vi "nanocal publish -- frontpanel.vi"(7 "publisher action":T3, 10 "nanocal data array IN":T1[](array[typedef])) -> (2 "nanocal data array OUT":T1[](array[typedef]))   [LabVIEW 2018]
uses:
  publisher action.ctl
  icicle.ctl
  nanocal-frontend -- data type.ctl
panel:
  out "nanocal data OUT":T2
  in  "nanocal data":T2
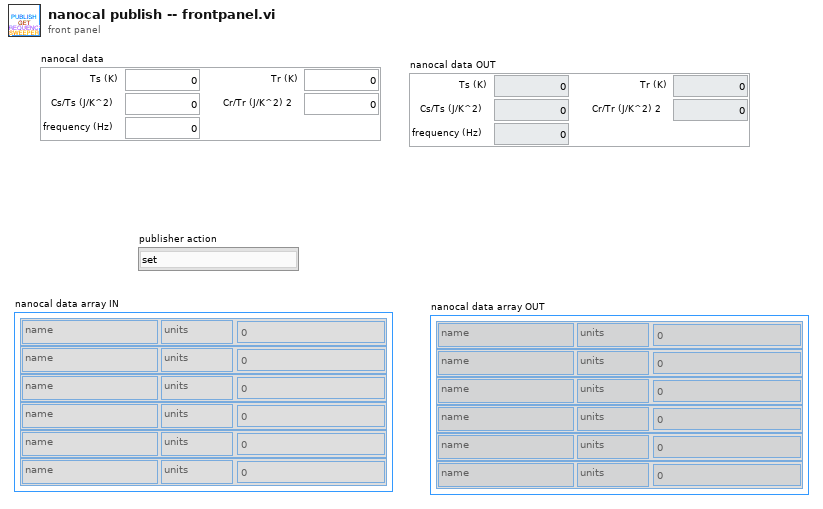
[diagram p1: front panel]
types:
  T1 = typedef "icicle.ctl" = cluster{"name":string, "units":string, "data":dbl}
  T2 = typedef "nanocal-frontend -- data type.ctl" = cluster{"frequency (Hz)":dbl, "Cs/Ts (J/K^2)":dbl, "Ts (K)":dbl, "Cr/Tr (J/K^2) 2":dbl, "Tr (K)":dbl}
  T3 = typedef "publisher action.ctl" = enum16{"set", "get", "init", "check"}
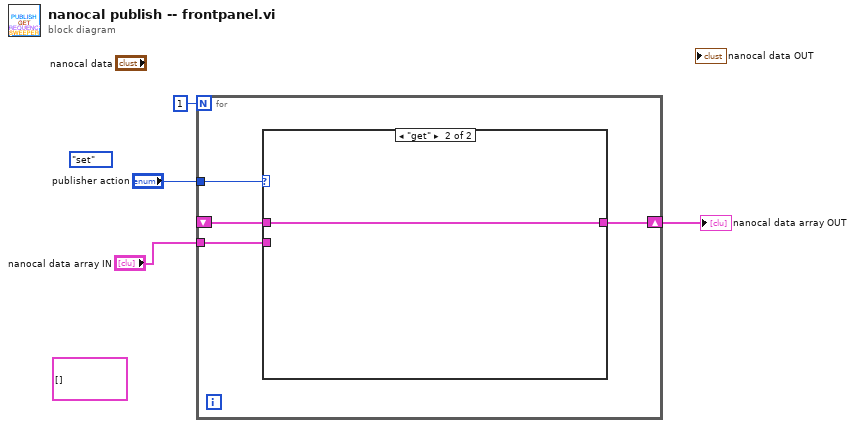
[diagram p0: block diagram]
diagram:
  (unwired) T1[] []
  (unwired) publisher_action."set" ("publisher action")
  n1 = for {
    N: 1 -> [_]
    tunnel: "publisher action" -> [w8]
    tunnel: "nanocal data array IN" -> [w6]
    shift-right: [w7] -> w1
    shift-left: _ -> [w5]
    n2 = case shown="\"get\"" w8 {
      tunnel: [w9 w10] -> w7
      tunnel: w6 -> [w9 _]
      tunnel: w5 -> [_ w10]
      frame "set", Default {
      }
      frame "get" {
      }
    }
  }
  "nanocal data array OUT" <- w1
